vi "ColorCell.vi"(6 "Cell Position":T1, 8 "error in (no error)":errorcluster, 9 "Table CtlRef In":refnum<vi>, 10 "Value":string, 11 "DigitalCol in":refnum<class "DigitalCol.lvclass">) -> (0 "error out":errorcluster, 1 "Table CtlRef Out":refnum<vi>, 3 "DigitalCol out":refnum<class "DigitalCol.lvclass">)   [LabVIEW 2013, in "DigitalCol.lvclass"]
doc: "Given cell value, set boolean coloring (unless cell is colored Disabled).\nGroupCol may override this if coloring of groups changes.\nThis VI is read-only w.r.t column data."
uses:
  DigitalCol.lvclass
  <vilib>/Utility/miscctls.llb/LVRowAndColumnTypeDef.ctl
  Column/Column.lvclass/Column.ctl
  Globals/DisabledColorGlobal.vi
  Column/Column.lvclass
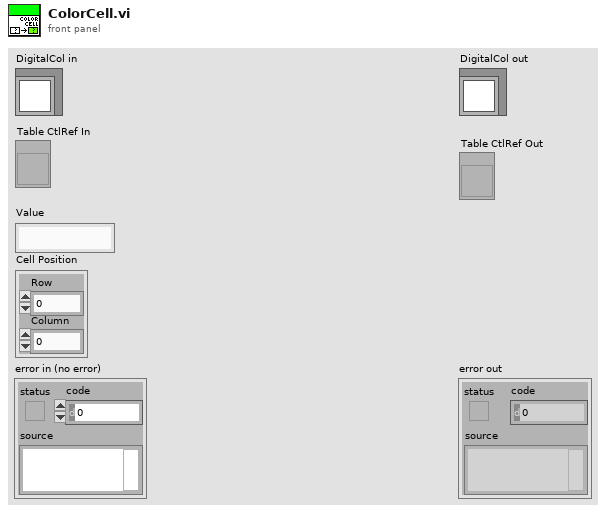
[diagram p1: front panel]
types:
  T1 = typedef "LVRowAndColumnTypeDef.ctl" = cluster{"Row":i32, "Column":i32}
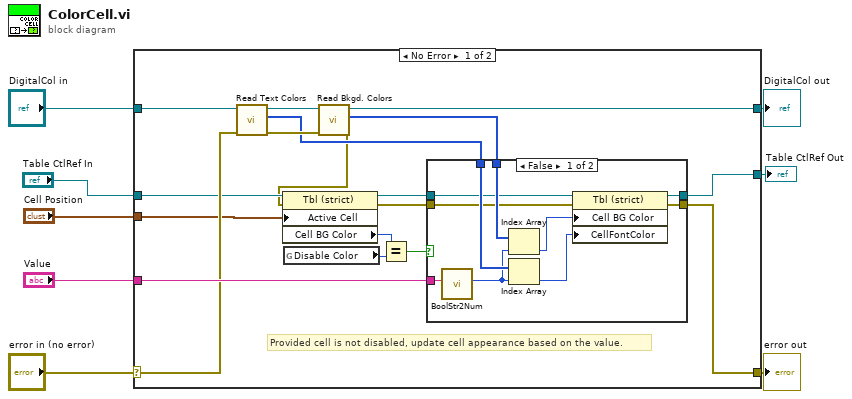
[diagram p0: block diagram]
diagram:
  n1 = case shown="No Error" "error in (no error)" {
    selector: "error in (no error)" -> [w19 w41]
    tunnel: [w18 w41] -> w7
    tunnel: [w21 w40] -> w5
    tunnel: "DigitalCol in" -> [w22 w40]
    tunnel: "Table CtlRef In" -> [w14 w39]
    tunnel: "Cell Position" -> [w10 _]
    tunnel: "Value" -> [w20 _]
    tunnel: [w17 w39] -> w1
    frame No Error {
      # "Provided cell is not disabled, update cell appearance based on the value."
      n2 = call "Read Text Colors.vi"("error in (no error)"=w19, "Column in"=w22) -> ("error out"=w25:errorcluster, "Text Colors"=w23:u32[], "Column out"=w26:refnum<class "DigitalCol.lvclass">)  [unwired: 7 in]
      n3 = global read "DisabledColorGlobal.vi" "Disable Color"() -> (w16:u32)
      n4 = call "Read Bkgd. Colors.vi"("error in (no error)"=w25, "Column in"=w26) -> ("error out"=w11:errorcluster, "Bkgd. Colors"=w24:u32[], "Column out"=w21:refnum<class "DigitalCol.lvclass">)  [unwired: 7 in]
      n5 = property class="Tbl (strict)"(reference=w14, error in=w11, "Active Cell"=w10) -> (reference out=w13:refnum<vi>, error out=w12:errorcluster, "Cell BG Color"=w15:u32)
      n6 = Equal?(x=w15, y=w16) -> (x = y?=w9:bool)
      n7 = case shown="False" w9 {
        tunnel: w24 -> [w36 _]
        tunnel: w23 -> [w34 _]
        tunnel: w20 -> [w31 _]
        tunnel: [w30 w37] -> w18
        tunnel: [w29 w38] -> w17
        tunnel: w13 -> [w28 w38]
        tunnel: w12 -> [w27 w37]
        frame False {
          n8 = call "BoolStr2Num.vi"("Boolean string"=w31) -> ("number"=w32:i32)  [unwired: 10 in]
          n9 = Index Array(array=w36, index=w32) -> (element=w35:u32)
          n10 = Index Array(array=w34, index=w32) -> (element=w33:u32)
          n11 = property class="Tbl (strict)"(reference=w28, error in=w27, "Cell BG Color"=w35, "CellFontColor"=w33) -> (reference out=w29:refnum<vi>, error out=w30:errorcluster)
        }
        frame True {
        }
      }
    }
    frame Error {
    }
  }
  "error out" <- w7
  "DigitalCol out" <- w5
  "Table CtlRef Out" <- w1
